vi "Periodic Random Noise.vi"(2 "seed":i32=-1, 3 "spectral amplitude":dbl=1.0 format="%0.2f", 4 "samples":i32=128) -> (0 "error":i32, 1 "periodic random noise":dbl[](array[numeric]))   [LabVIEW 2020, in "NI_AALBase.lvlib"]
doc: "Generates an array containing periodic random noise (PRN)."
uses:
  <vilib>/Analysis/NI_AALBase.lvlib
  <resource>/lvanlys.dll
panel:
  # "Periodic Random Noise"
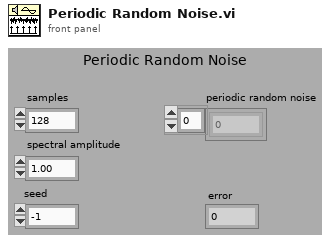
[diagram p1: front panel]
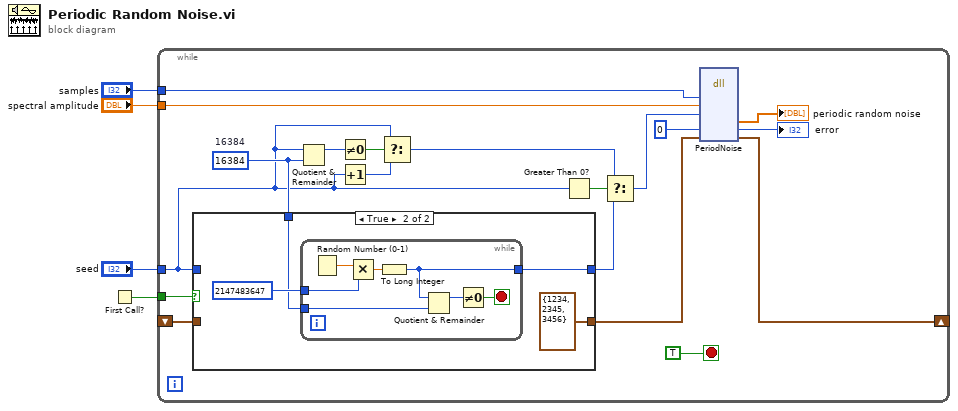
[diagram p0: block diagram]
diagram:
  n1 = First Call?() -> (First Call?: T/F=w4:bool)
  n2 = while {
    shift-right: [w19] -> _
    shift-left: _ -> [w6]
    tunnel: w4 -> [w5]
    tunnel: "spectral amplitude" -> [w21]
    tunnel: "samples" -> [w20]
    tunnel: "seed" -> [w7]
    stop <- TRUE stop-if-true
    w16 = 16384  # 16384
    n3 = case shown="True" w5 {
      tunnel: w6 -> [w25 _]
      tunnel: [w25 cluster{"xSeed":i32, "ySeed":i32, "zSeed":i32} {"xSeed"=1234, "ySeed"=2345, "zSeed"=3456} ("RNGState")] -> w9
      tunnel: [w24 w26] -> w15
      tunnel: w7 -> [w24 _]
      tunnel: w16 -> [_ w27]
      frame False {
      }
      frame True {
        n4 = while {
          tunnel: [w34] -> w26
          tunnel: w27 -> [w33]
          tunnel: 2147483647 ("x") -> [w30]
          stop <- w31 stop-if-true
          n5 = Random Number (0-1)() -> (number: 0 to 1=w35:dbl)
          n6 = Multiply(x=w35, y=w30) -> (x*y=w36:dbl)
          n7 = To Long Integer(number=w36) -> (32bit integer=w34:i32)
          n8 = Quotient & Remainder(x=w34, y=w33) -> (x-y*floor(x/y)=w32:i32)  [unwired: 1 out]
          n9 = Not Equal To 0?(x=w32) -> (x != 0?=w31:bool)
        }
      }
    }
    n10 = Quotient & Remainder(x=w7, y=w16) -> (x-y*floor(x/y)=w11:i32)  [unwired: 1 out]
    n11 = Not Equal To 0?(x=w11) -> (x != 0?=w12:bool)
    n12 = Increment(x=w7) -> (x+1=w13:i32)
    n13 = Select(t=w7, s=w12, f=w13) -> (s? t:f=w14:i32)
    n14 = Greater Than 0?(x=w7) -> (x > 0?=w10:bool)
    n15 = Select(t=w14, s=w10, f=w15) -> (s? t:f=w8:i32)
    n16 = dll-call lib="e:/builds/penguin/labview/branches/2020/dev/dist/resource/lvanlys.*" fn="PeriodNoise"("samples"=w20, "spectral amplitude"=w21, "seed"=w8, "error"=0, "RNGState"=w9) -> ("periodic random noise"=→"periodic random noise":dbl[], "error"=→"error":i32, "RNGState"=w19:cluster{"xSeed":i32, "ySeed":i32, "zSeed":i32})  [unwired: 8 in, 2 out]
  }
